vi "Disconnect.vi"(8 "error in":errorcluster, 11 "Thorlabs In":refnum<class "Thorlabs.lvclass">) -> (0 "error out":errorcluster, 3 "Thorlabs Out":refnum<class "Thorlabs.lvclass">)   [LabVIEW 2018, in "Thorlabs.lvlib" / "Thorlabs.lvclass"]
doc: "This VI calls Disconnect on the Device. It then destroys the reference.\n\nCreator: Slade Jeppesen\nCreated Date: 09/29/20"
uses:
  Thorlabs.lvclass
  Thorlabs.lvclass/Thorlabs.ctl
  C:/AME Test Engineering/LabVIEW/PPLs/Axis/DLLs/ThorLabs.MotionControl.KCube.DCServoCLI.dll
  PPLs/Axis/DLLs/ThorLabs.MotionControl.KCube.DCServoCLI.dll
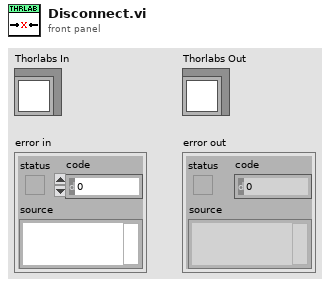
[diagram p1: front panel]
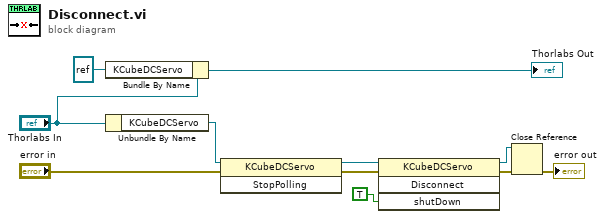
[diagram p0: block diagram]
diagram:
  n1 = Bundle By Name(cluster="Thorlabs In", "KCubeDCServo"=refnum<k24> refnum) -> (→"Thorlabs Out":refnum<class "Thorlabs.lvclass">)
  n2 = Unbundle By Name("Thorlabs In") -> ("KCubeDCServo"=w3:refnum<k24>)
  n3 = invoke class="KCubeDCServo" method="StopPolling"(reference=w3, error in="error in") -> (reference out=w2:refnum<k24>, error out=w4:errorcluster)  [unwired: 1 in, 1 out]
  n4 = invoke class="KCubeDCServo" method="Disconnect"(reference=w2, error in=w4, "shutDown"=TRUE) -> (reference out=w9:refnum<k24>, error out=w8:errorcluster)  [unwired: 1 in, 2 out]
  n5 = Close Reference(reference=w9, error in (no error)=w8) -> (error out=→"error out":errorcluster)
